vi "Poll.Main.vi"(10 "Paramaters":variant, 11 "Process":refnum<class "Process.lvclass">) -> ()   [LabVIEW 2019, in "OPC UA Client Addon Engine.lvlib"]
uses:
  OPC UA Client Addon Engine.lvlib
  <vilib>/OPCUA/NI OPC UA Client.lvlib
  Addon Shared/DataRefs.Location.ctl
  Addon Shared/OPC UA Client Addon Shared.lvlib
  <vilib>/NI/NIVS Inline Async API/_VS Inline Async API/Process/Process.lvclass
  Addon Shared/OPCConnection.Properties.ctl
  Addon Shared/Poll.ListProperties.ctl
  <vilib>/NI VeriStand/Custom Device API/Data Reference.ctl
  <vilib>/NI VeriStand/Custom Device API/Custom Device API.lvlib
  Addon Shared/Tag.WriteProperties.Info.ctl
  Addon Shared/Tags.ReadWriteRefs.ctl
  Addon Shared/Compiled.Settings.ctl
  <vilib>/NI VeriStand/Custom Device API/Custom Device Target Type.ctl
  Types/Poll.Parameters.ctl
  <vilib>/NI/NIVS Inline Async API/_Data Access Engine/Data Access Engine/Data Access Engine.lvclass
  <vilib>/NI/NIVS Inline Async API/_Data Access Engine/Data Access Engine/Methods/Write.Data.vi
  <vilib>/OPCUA/client/internal/Write Int64.vi
  <vilib>/OPCUA/client/internal/Write Int32.vi
  <vilib>/OPCUA/client/internal/Write UInt16.vi
  <vilib>/OPCUA/client/internal/Write Byte.vi
  <vilib>/OPCUA/client/internal/Write Int32 Array.vi
  <vilib>/OPCUA/client/internal/Write Bool Array.vi
  <vilib>/OPCUA/client/internal/Write SByte Array.vi
  <vilib>/OPCUA/client/internal/Write Int16.vi
  <vilib>/OPCUA/client/internal/Write SByte.vi
  <vilib>/OPCUA/client/internal/Write DateTime.vi
  <vilib>/OPCUA/client/internal/Write Bool.vi
  <vilib>/OPCUA/client/internal/Write UInt64 Array.vi
  <vilib>/OPCUA/client/internal/Write Float Array.vi
  <vilib>/OPCUA/client/internal/Write UInt64.vi
  <vilib>/OPCUA/client/internal/Write Int16 Array.vi
  <vilib>/OPCUA/client/internal/Write UInt16 Array.vi
  <vilib>/OPCUA/client/internal/Write Byte Array.vi
  <vilib>/OPCUA/client/internal/Write UInt32 Array.vi
  <vilib>/OPCUA/client/internal/Write DateTime Array.vi
  <vilib>/OPCUA/client/internal/Write Float.vi
  <vilib>/OPCUA/client/internal/Write Double Array.vi
  <vilib>/OPCUA/client/internal/Write UInt32.vi
  <vilib>/OPCUA/client/internal/Write Double.vi
  <vilib>/OPCUA/client/internal/Write Int64 Array.vi
panel:
  out "Read Code":i32
  out "Write Code":i32
  out "Read Table":variant
  out "Write Table":variant
  in  "error in (no error)":errorcluster
  out "error out":errorcluster
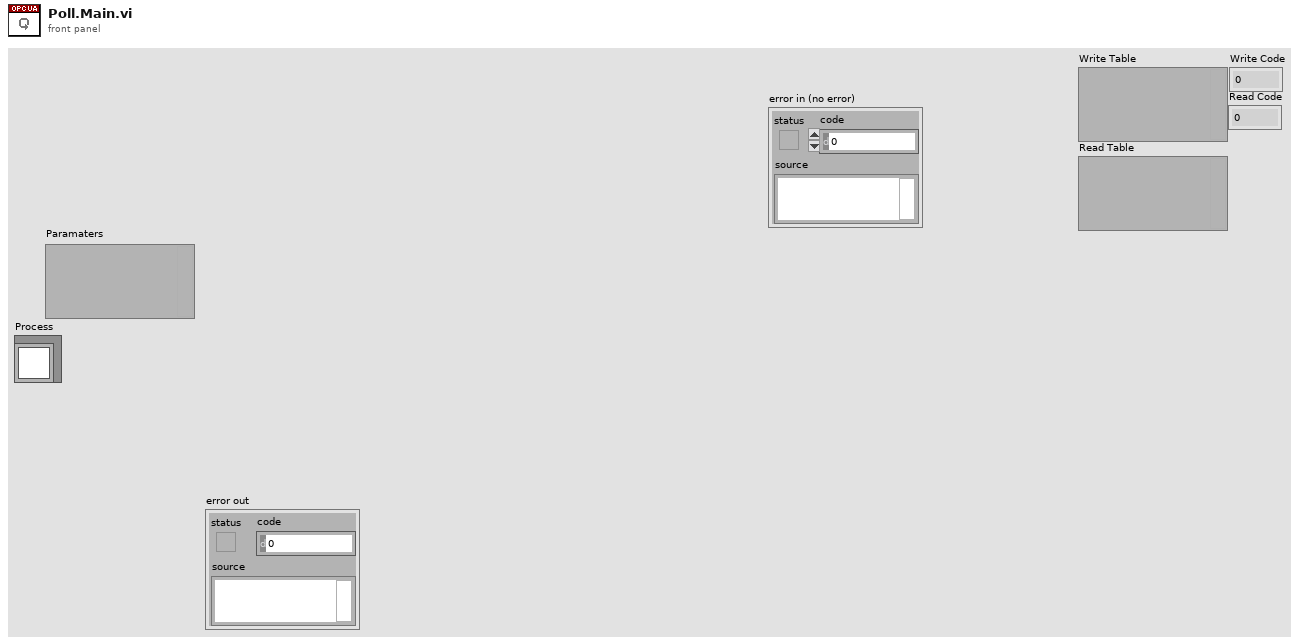
[diagram p1: front panel]
types:
  T1 = typedef "OPC UA Client Addon Engine.lvlib/Poll.Parameters.ctl" = cluster{"Name":string, "Settings":T2, "WriteData":refnum<k33>, "ReadData":refnum<k33>, "WriteUpdate":refnum<k33>, "ReadUpdate":refnum<k33>}
  T2 = typedef "OPC UA Client Addon Shared.lvlib/Compiled.Settings.ctl" = cluster{"Connection.Properties":T3, "PollEngine.Settings":T4[], "LUT":variant, "Write Locations":T5[], "TotalTags":u32, "Data Refs":T6, "Target Type":T8}
  T3 = typedef "OPC UA Client Addon Shared.lvlib/OPCConnection.Properties.ctl" = cluster{"Server IP Address":string, "Server Port":u16, "Message Mode":enum16{"None", "Sign", "Sign and Encrypt"}, "Security":enum16{"Basic256", "Basic128Rsa15"}, "User Name":string, "Password":string, "Client Certificate":path, "Server Certificate":path, "Server Certificate (RT)":path, "Client Certificate (RT)":path}
  T4 = typedef "OPC UA Client Addon Shared.lvlib/Poll.ListProperties.ctl" = cluster{"Poll Rate":dbl, "Tags":string[]}
  T5 = typedef "OPC UA Client Addon Shared.lvlib/Tag.WriteProperties.Info.ctl" = cluster{"Path":string, "Offset":i32, "Length":i32, "DataType":u32}
  T6 = typedef "OPC UA Client Addon Shared.lvlib/Tags.ReadWriteRefs.ctl" = cluster{"Read Refs":T7[], "Read Values":dbl[], "Read?":bool[], "Access":enum8{"Null", "Read", "Write", "Read&Write"}[], "Write Refs":T7[], "Write Values":dbl[], "Write?":bool[], "Write Only Location":u32, "Write? Reset":bool[]}
  T7 = typedef "Custom Device API.lvlib/Data Reference.ctl" = i32
  T8 = typedef "Custom Device API.lvlib/Custom Device Target Type.ctl" = enum16{"PharLap", "VxWorks", "Windows", "Linux_32_ARM", "Linux_x64"}
  T9 = typedef "OPC UA Client Addon Shared.lvlib/DataRefs.Location.ctl" = cluster{"Offset":i32, "Length":i32}
  T10 = typedef "OPC UA Client Addon Engine.lvlib/Poll.StateVariables.ctl" = cluster{"SubscriptionIDs":u32[], "OPCEvent":refnum<event-registration>, "Stop Ref":refnum<data-value>, "OPC UA client Ref":refnum<k21>, "Data Change":refnum<user-event>, "Process":refnum<class "Process.lvclass">, "Status Ref":T11}
  T11 = typedef "Data Access Engine.lvlib/Data Access Engine.lvclass/Write.DVR.ctl" = refnum<data-value>
  T12 = typedef "Subscription Data Change.ctl" = cluster{"node ID":T13, " value":variant, "timestamp":timestamp, "data type":T14, "status code":T15}
  T13 = typedef "NodeId.ctl" = string
  T14 = typedef "Data Type.ctl" = u16
  T15 = typedef "OPC UA StatusCode.ctl" = u32
  T16 = typedef "Subscription ID.ctl" = u32
  T17 = typedef "OPC UA Client Refnum.ctl" = refnum<k21>
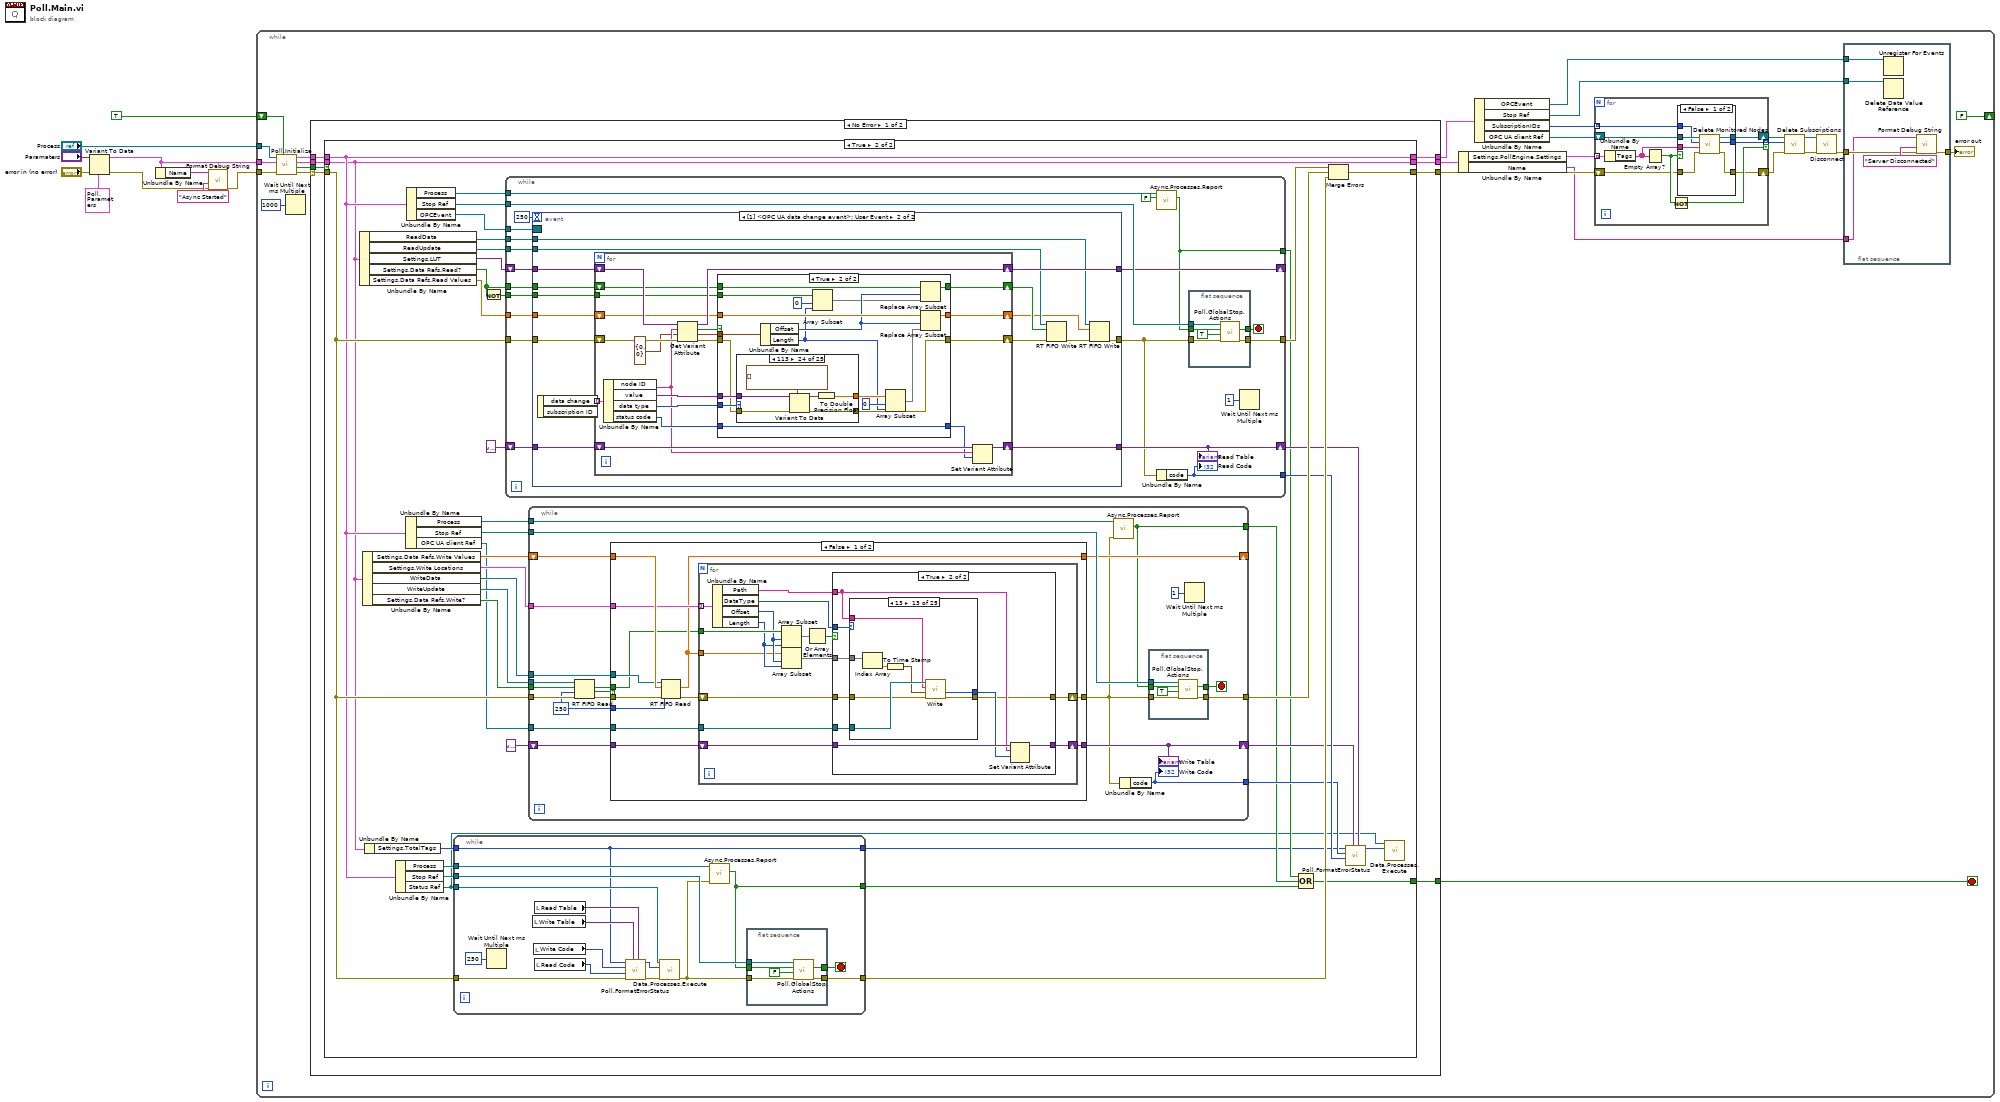
[diagram p0: block diagram]
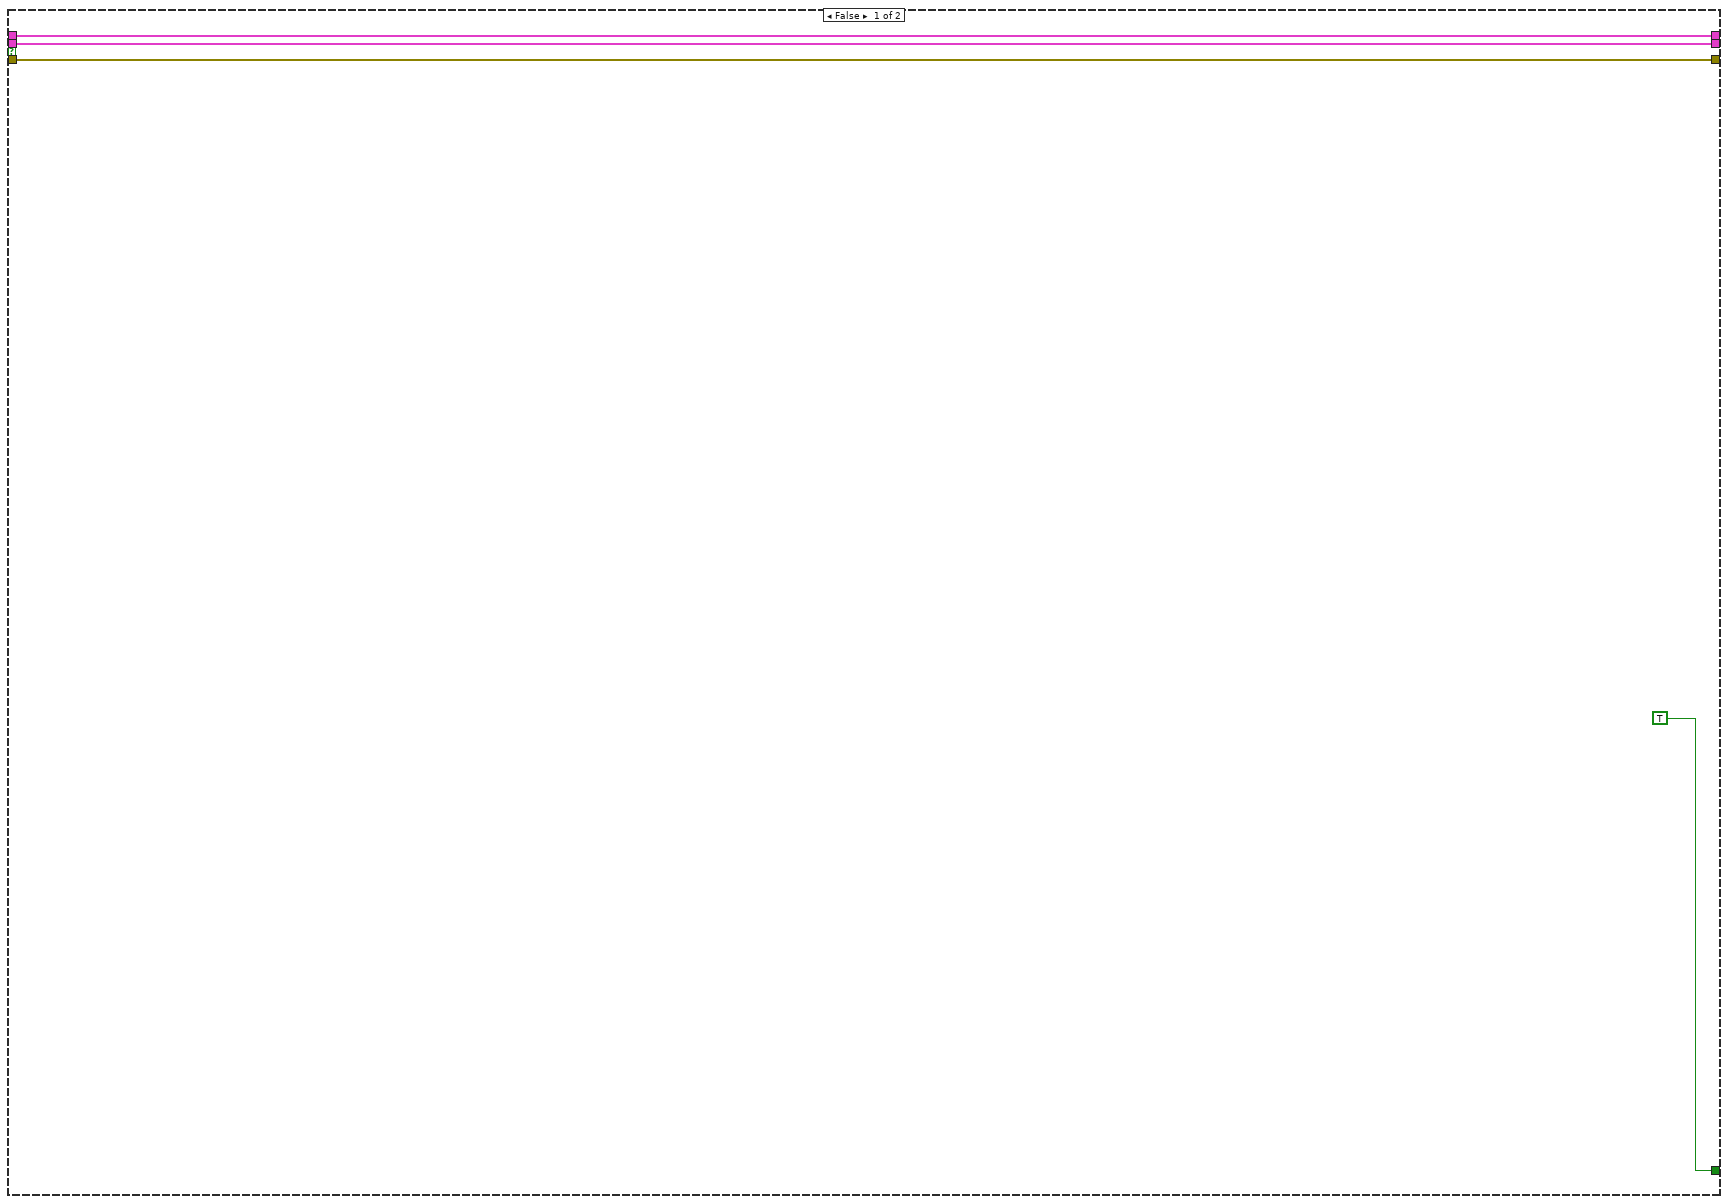
[diagram p3: hidden frame]
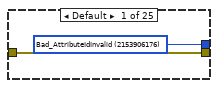
[diagram p5: hidden frame]
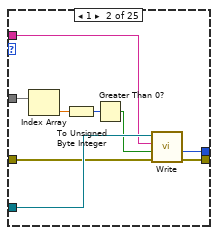
[diagram p6: hidden frame]
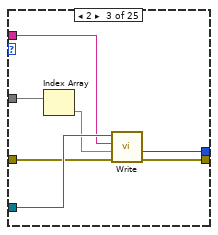
[diagram p7: hidden frame]
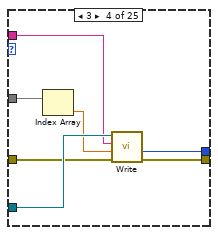
[diagram p8: hidden frame]
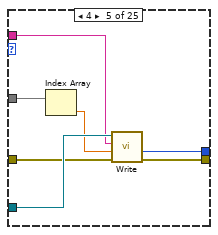
[diagram p9: hidden frame]
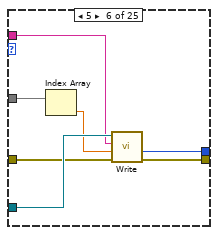
[diagram p10: hidden frame]
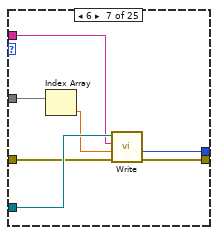
[diagram p11: hidden frame]
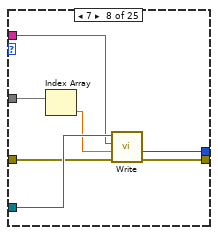
[diagram p12: hidden frame]
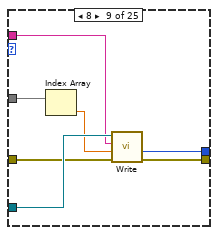
[diagram p13: hidden frame]
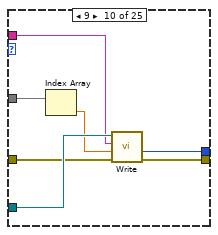
[diagram p14: hidden frame]
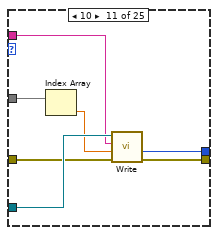
[diagram p15: hidden frame]
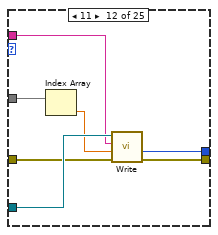
[diagram p16: hidden frame]
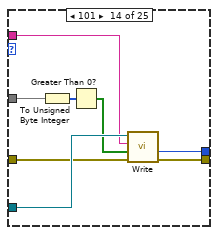
[diagram p17: hidden frame]
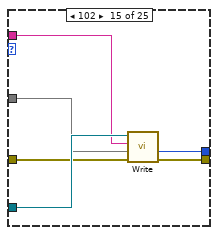
[diagram p18: hidden frame]
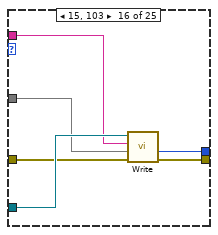
[diagram p19: hidden frame]
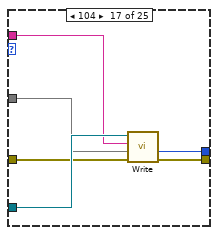
[diagram p20: hidden frame]
diagram:
  n1 = Variant To Data(error in="error in (no error)", type=T1 {"Name"="", "Settings"={"Connection.Properties"={"Server IP Address"="", "Server Port"=0, "Message Mode"=enum."None", "Security"=enum."Basic256", "User Name"="", "Password"="", "Client Certificate"=path "", "Server Certificate"=path "", "Server Certificate (RT)"=path "", "Client Certificate (RT)"=path ""}, "PollEngine.Settings"=[], "LUT"=variant, "Write Locations"=[], "TotalTags"=0, "Data Refs"={"Read Refs"=[], "Read Values"=[], "Read?"=[], "Access"=[], "Write Refs"=[], "Write Values"=[], "Write?"=[], "Write Only Location"=0, "Write? Reset"=[]}, "Target Type"=enum."PharLap"}, "WriteData"=refnum, "ReadData"=refnum, "WriteUpdate"=refnum, "ReadUpdate"=refnum} ("Parameters"), Variant="Paramaters") -> (data=w5:T1, error out=w2:errorcluster)
  n2 = Unbundle By Name(w5) -> ("Name"=w3:string)
  n3 = call "Format Debug String.vi"("error in (no error)"=w2, "State"="Async Started", "Name"=w3) -> ("error out"=w1:errorcluster)  [unwired: 8 in]
  n4 = while {
    tunnel: w1 -> [w32]
    tunnel: w5 -> [w31]
    shift-right: [FALSE] -> _
    shift-left: TRUE -> [w30]
    tunnel: "Process" -> [w27]
    stop <- w28 stop-if-true
    n5 = call "Poll.Initialize.vi"("FirstCall?"=w30, "error in (no error)"=w32, "Parameters in"=w31, "Process"=w27) -> ("error out"=w34:errorcluster, "notification"=w36:bool, "Parameters out"=w37:T1, "Settings"=w35:T10)  [unwired: 4 in]
    n6 = Wait Until Next ms Multiple(millisecond multiple=u32 1000) -> ()  [unwired: 1 out]
    n7 = case shown="No Error" w34 {
      selector: w34 -> [w67 w619]
      tunnel: [w63 w619] -> w26
      tunnel: w37 -> [w70 w623]
      tunnel: w36 -> [w69 _]
      tunnel: w35 -> [w68 w621]
      tunnel: [w65 w623] -> w25
      tunnel: [w64 w621] -> w24
      tunnel: [w66 w618] -> w28
      frame No Error {
        n8 = case shown="True" w69 {
          tunnel: w68 -> [w73 w112]
          tunnel: w67 -> [w74 w114]
          tunnel: [w74 w113] -> w63
          tunnel: w70 -> [w72 w111]
          tunnel: [w73 w112] -> w64
          tunnel: [w72 w111] -> w65
          tunnel: [TRUE w78] -> w66
          frame False {
          }
          frame True {
            n9 = Unbundle By Name(w111) -> ("ReadData"=w104:refnum<k33>, "ReadUpdate"=w91:refnum<k33>, "Settings.LUT"=w103:variant, "Settings.Data Refs.Read?"=w90:bool[], "Settings.Data Refs.Read Values"=w88:dbl[])
            n10 = Unbundle By Name(w111) -> ("Settings.Data Refs.Write Values"=w107:dbl[], "Settings.Write Locations"=w106:T5[], "WriteData"=w105:refnum<k33>, "WriteUpdate"=w93:refnum<k33>, "Settings.Data Refs.Write?"=w92:bool[])
            n11 = Unbundle By Name(w111) -> ("Settings.TotalTags"=w77:u32)
            n12 = Unbundle By Name(w112) -> ("Process"=w96:refnum<class "Process.lvclass">, "Stop Ref"=w99:refnum<data-value>, "Status Ref"=w76:T11)
            n13 = Unbundle By Name(w112) -> ("Process"=w95:refnum<class "Process.lvclass">, "Stop Ref"=w100:refnum<data-value>, "OPC UA client Ref"=w87:refnum<k21>)
            n14 = Unbundle By Name(w112) -> ("Process"=w94:refnum<class "Process.lvclass">, "Stop Ref"=w101:refnum<data-value>, "OPCEvent"=w102:refnum<event-registration>)
            n15 = while {
              tunnel: w114 -> [w130]
              tunnel: w99 -> [w129]
              tunnel: [w126] -> w98
              tunnel: w96 -> [w125]
              tunnel: [w117] -> w81
              tunnel: w76 -> [w116]
              tunnel: w77 -> [w115]
              tunnel: [w115] -> w75
              stop <- w119 stop-if-true
              n16 = Wait Until Next ms Multiple(millisecond multiple=u32 250) -> ()  [unwired: 1 out]
              n17 = local read "Write Table"() -> (w121:variant)
              n18 = local read "Write Code"() -> (w124:i32)
              n19 = local read "Read Table"() -> (w120:variant)
              n20 = local read "Read Code"() -> (w123:i32)
              n21 = call "Poll.FormatErrorStatus.vi"("Read Table"=w120, "Write Table"=w121, "error in (no error)"=w130, "Read Code"=w123, "Write Code"=w124, "TotalTags"=w115) -> ("error out"=w128:errorcluster, "ErrorStatus"=w127:u32[])  [unwired: 4 in]
              n22 = call-poly <vilib>:"Data.Processes.Execute.vi"("error in (no error)"=w128, "Values"=w127, "Ref"=w116) -> ("error out"=w118:errorcluster)  [unwired: 8 in]
              n23 = call <vilib>:"Async.Processes.Report.vi"("Error"=w118, "Process in"=w125) -> ("Stop"=w117:bool)  [unwired: 8 in, 1 out]
              n24 = flat-sequence {
                tunnel: w129 -> [w135]
                tunnel: [w134] -> w119
                tunnel: w118 -> [w133]
                tunnel: [w132] -> w126
                tunnel: w117 -> [w131]
                frame #0 {
                  n25 = call "Poll.GlobalStop.Actions.vi"("error in (no error)"=w133, "Stop on Error?"=FALSE, "Stop?"=w131, "Stop Ref"=w135) -> ("error out"=w132:errorcluster, "Latched Stop"=w134:bool)  [unwired: 5 in, 1 out]
                }
              }
            }
            n26 = Not(x=w90) -> (.not. x?=w89:bool[])
            n27 = while {
              tunnel: w102 -> [w390]
              shift-right: [w384] -> _
              shift-left: w103 -> [w387]
              tunnel: w104 -> [w379]
              tunnel: w114 -> [w388]
              tunnel: [w381] -> w97
              shift-right: [w383] -> w85
              shift-left: variant ("variant") -> [w386]
              tunnel: w101 -> [w385]
              tunnel: w94 -> [w380]
              tunnel: w91 -> [w378]
              tunnel: w90 -> [w377]
              tunnel: w89 -> [w376]
              tunnel: [w374] -> w84
              tunnel: w88 -> [w375]
              tunnel: [w371] -> w79
              stop <- w373 stop-if-true
              n28 = event shown="[1] <OPC UA data change event>: User Event" {
                selector: w390 -> [_ _]
                dyn-events: _ -> [_ _]
                timeout: 250 -> [_ _]
                tunnel: w388 -> [w399 w412]
                tunnel: [w399 w408] -> w370
                tunnel: w387 -> [w398 w414]
                tunnel: [w398 w413] -> w384
                tunnel: w386 -> [w397 w411]
                tunnel: [w397 w410] -> w383
                tunnel: w375 -> [_ w409]
                tunnel: w379 -> [_ w407]
                tunnel: w378 -> [_ w404]
                tunnel: w377 -> [_ w402]
                tunnel: w376 -> [_ w401]
                event Timeout {
                  n29 = event-data() -> ()  [unwired: 1 in, 2 out]
                }
                event User Event {
                  n30 = event-data() -> ("data change"=w415:T12[])  [unwired: 1 in, 1 out]
                  n31 = for {
                    tunnel: w415 -> [w436] mode=indexing
                    shift-right: [w432] -> w413
                    shift-left: w414 -> [w434]
                    shift-right: [w416] -> w406
                    shift-left: w412 -> [w431]
                    shift-right: [w423] -> w410
                    shift-left: w411 -> [w426]
                    shift-right: [w420] -> w400
                    shift-left: w409 -> [w421]
                    shift-right: [w418] -> w403
                    shift-left: w402 -> [w419]
                    tunnel: w401 -> [w417]
                    n32 = Unbundle By Name(w436) -> ("node ID"=w425:T13, "value"=w435:variant, "data type"=w430:T14, "status code"=w428:T15)
                    n33 = Get Variant Attribute(Variant=w434, name=w425, default value (empty Variant)=T9 {"Offset"=0, "Length"=0} ("cluster"), error in=w431) -> (duplicate Variant=w432:variant, found=w427:bool, value=w433:T9, error out=w429:errorcluster)
                    n34 = case shown="True" w427 {
                      tunnel: w435 -> [_ w458]
                      tunnel: w433 -> [_ w453]
                      tunnel: [w440 w452] -> w416
                      tunnel: w430 -> [_ w457]
                      tunnel: w429 -> [w440 w456]
                      tunnel: w428 -> [_ w455]
                      tunnel: [w439 w455] -> w424
                      tunnel: w421 -> [w438 w454]
                      tunnel: [w438 w449] -> w420
                      tunnel: w419 -> [w437 w445]
                      tunnel: [w437 w446] -> w418
                      tunnel: w417 -> [_ w442]
                      frame False {
                        w439 = u32 2153906176 items=["Good"=0, "Bad_AttributeIdInvalid"=2153906176, "Bad_BrowseDirectionInvalid"=2152529920, "Bad_BrowseNameInvalid"=2153775104, "Bad_ContentFilterInvalid"=2152202240, "Bad_ContinuationPointInvalid"=2152333312, "Bad_DataEncodingInvalid"=2151153664, "Bad_DataEncodingUnsupported"=2151219200, "Bad_EventFilterInvalid"=2152136704, "Bad_FilterNotAllowed"=2152005632, "Bad_FilterOperandInvalid"=2160132096, "Bad_HistoryOperationInvalid"=2154889216, "Bad_HistoryOperationUnsupported"=2154954752, "Bad_IndexRangeInvalid"=2151022592, "Bad_IndexRangeNoData"=2151088128, "Bad_MonitoredItemFilterInvalid"=2151874560, "Bad_MonitoredItemFilterUnsupported"=2151940096, "Bad_MonitoredItemIdInvalid"=2151809024, "Bad_MonitoringModeInvalid"=2151743488, "Bad_NoCommunication"=2150694912, "Bad_NoContinuationPoints"=2152398848, "Bad_NodeClassInvalid"=2153709568, "Bad_NodeIdInvalid"=2150825984, "Bad_NodeIdUnknown"=2150891520, "Bad_NoDeleteRights"=2154364928, "Bad_NodeNotInView"=2152595456, "Bad_NotFound"=2151546880, "Bad_NotImplemented"=2151677952, "Bad_NotReadable"=2151284736, "Bad_NotSupported"=2151481344, "Bad_NotWritable"=2151350272, "Bad_ObjectDeleted"=2151612416, "Bad_OutOfRange"=2151415808, "Bad_ReferenceTypeIdInvalid"=2152464384, "Bad_SourceNodeIdInvalid"=2154037248, "Bad_StructureMissing"=2152071168, "Bad_TargetNodeIdInvalid"=2154102784, "Bad_TypeDefinitionInvalid"=2153971712, "Bad_TypeMismatch"=2155085824, "Bad_WaitingForInitialData"=2150760448] ("status")
                      }
                      frame True {
                        n35 = case shown="113" w457 {
                          tunnel: w458 -> [w466 w473 w480 w487 w494 w501 w508 w515 w522 w529 w536 w543 w550 w556 w562 w568 w574 w580 w586 w592 w598 w604 w610 w616 _]
                          tunnel: w456 -> [w465 w472 w479 w486 w493 w500 w507 w514 w521 w528 w535 w542 w549 w555 w561 w567 w573 w579 w585 w591 w597 w603 w609 w615 w617]
                          tunnel: [w464 w471 w478 w485 w492 w499 w506 w513 w520 w527 w534 w541 w548 w554 w560 w566 w572 w578 w584 w590 w596 w602 w608 w614 w617] -> w452
                          tunnel: [w459 w468 w475 w482 w489 w496 w503 w510 w517 w524 w531 w538 w544 w552 w558 w564 w570 w576 w582 w588 w594 w600 w606 w612 _] -> w451
                          frame 1 {
                            n36 = Variant To Data(error in=w465, type=FALSE, Variant=w466) -> (data=w462:bool, error out=w464:errorcluster)
                            n37 = Boolean To (0,1)(Boolean=w462) -> (0, 1=w461:i16)
                            n38 = To Double Precision Float(number=w461) -> (double precision float=w460:dbl)
                            n39 = Build Array(w460) -> (w459:dbl[])
                          }
                          frame 2 {
                            n40 = Variant To Data(error in=w472, type=i8 0, Variant=w473) -> (data=w467:i8, error out=w471:errorcluster)
                            n41 = To Double Precision Float(number=w467) -> (double precision float=w469:dbl)
                            n42 = Build Array(w469) -> (w468:dbl[])
                          }
                          frame 3 {
                            n43 = Variant To Data(error in=w479, type=u8 0, Variant=w480) -> (data=w474:u8, error out=w478:errorcluster)
                            n44 = To Double Precision Float(number=w474) -> (double precision float=w476:dbl)
                            n45 = Build Array(w476) -> (w475:dbl[])
                          }
                          frame 4 {
                            n46 = Variant To Data(error in=w486, type=i16 0, Variant=w487) -> (data=w481:i16, error out=w485:errorcluster)
                            n47 = To Double Precision Float(number=w481) -> (double precision float=w483:dbl)
                            n48 = Build Array(w483) -> (w482:dbl[])
                          }
                          frame 5 {
                            n49 = Variant To Data(error in=w493, type=u16 0, Variant=w494) -> (data=w488:u16, error out=w492:errorcluster)
                            n50 = To Double Precision Float(number=w488) -> (double precision float=w490:dbl)
                            n51 = Build Array(w490) -> (w489:dbl[])
                          }
                          frame 6 {
                            n52 = Variant To Data(error in=w500, type=0, Variant=w501) -> (data=w495:i32, error out=w499:errorcluster)
                            n53 = To Double Precision Float(number=w495) -> (double precision float=w497:dbl)
                            n54 = Build Array(w497) -> (w496:dbl[])
                          }
                          frame 7 {
                            n55 = Variant To Data(error in=w507, type=u32 0, Variant=w508) -> (data=w502:u32, error out=w506:errorcluster)
                            n56 = To Double Precision Float(number=w502) -> (double precision float=w504:dbl)
                            n57 = Build Array(w504) -> (w503:dbl[])
                          }
                          frame 8 {
                            n58 = Variant To Data(error in=w514, type=i64 0, Variant=w515) -> (data=w509:i64, error out=w513:errorcluster)
                            n59 = To Double Precision Float(number=w509) -> (double precision float=w511:dbl)
                            n60 = Build Array(w511) -> (w510:dbl[])
                          }
                          frame 9 {
                            n61 = Variant To Data(error in=w521, type=u64 0, Variant=w522) -> (data=w516:u64, error out=w520:errorcluster)
                            n62 = To Double Precision Float(number=w516) -> (double precision float=w518:dbl)
                            n63 = Build Array(w518) -> (w517:dbl[])
                          }
                          frame 10 {
                            n64 = Variant To Data(error in=w528, type=sgl 0.0, Variant=w529) -> (data=w523:sgl, error out=w527:errorcluster)
                            n65 = To Double Precision Float(number=w523) -> (double precision float=w525:dbl)
                            n66 = Build Array(w525) -> (w524:dbl[])
                          }
                          frame 11 {
                            n67 = Variant To Data(error in=w535, type=0.0, Variant=w536) -> (data=w530:dbl, error out=w534:errorcluster)
                            n68 = To Double Precision Float(number=w530) -> (double precision float=w532:dbl)
                            n69 = Build Array(w532) -> (w531:dbl[])
                          }
                          frame 13 {
                            n70 = Variant To Data(error in=w542, type=timestamp(0 s since 1904-01-01), Variant=w543) -> (data=w537:timestamp, error out=w541:errorcluster)
                            n71 = To Double Precision Float(number=w537) -> (double precision float=w539:dbl)
                            n72 = Build Array(w539) -> (w538:dbl[])
                          }
                          frame 101 {
                            n73 = Variant To Data(error in=w549, type=bool[] [], Variant=w550) -> (data=w547:bool[], error out=w548:errorcluster)
                            n74 = Boolean To (0,1)(Boolean=w547) -> (0, 1=w546:i16[])
                            n75 = To Double Precision Float(number=w546) -> (double precision float=w544:dbl[])
                          }
                          frame 102 {
                            n76 = Variant To Data(error in=w555, type=i8[] [], Variant=w556) -> (data=w551:i8[], error out=w554:errorcluster)
                            n77 = To Double Precision Float(number=w551) -> (double precision float=w552:dbl[])
                          }
                          frame 15, 103 {
                            n78 = Variant To Data(error in=w561, type=u8[] [], Variant=w562) -> (data=w557:u8[], error out=w560:errorcluster)
                            n79 = To Double Precision Float(number=w557) -> (double precision float=w558:dbl[])
                          }
                          frame 104 {
                            n80 = Variant To Data(error in=w567, type=i16[] [], Variant=w568) -> (data=w563:i16[], error out=w566:errorcluster)
                            n81 = To Double Precision Float(number=w563) -> (double precision float=w564:dbl[])
                          }
                          frame 105 {
                            n82 = Variant To Data(error in=w573, type=u16[] [], Variant=w574) -> (data=w569:u16[], error out=w572:errorcluster)
                            n83 = To Double Precision Float(number=w569) -> (double precision float=w570:dbl[])
                          }
                          frame 106 {
                            n84 = Variant To Data(error in=w579, type=i32[] [], Variant=w580) -> (data=w575:i32[], error out=w578:errorcluster)
                            n85 = To Double Precision Float(number=w575) -> (double precision float=w576:dbl[])
                          }
                          frame 107 {
                            n86 = Variant To Data(error in=w585, type=u32[] [], Variant=w586) -> (data=w581:u32[], error out=w584:errorcluster)
                            n87 = To Double Precision Float(number=w581) -> (double precision float=w582:dbl[])
                          }
                          frame 108 {
                            n88 = Variant To Data(error in=w591, type=i64[] [], Variant=w592) -> (data=w587:i64[], error out=w590:errorcluster)
                            n89 = To Double Precision Float(number=w587) -> (double precision float=w588:dbl[])
                          }
                          frame 109 {
                            n90 = Variant To Data(error in=w597, type=u64[] [], Variant=w598) -> (data=w593:u64[], error out=w596:errorcluster)
                            n91 = To Double Precision Float(number=w593) -> (double precision float=w594:dbl[])
                          }
                          frame 110 {
                            n92 = Variant To Data(error in=w603, type=sgl[] [], Variant=w604) -> (data=w599:sgl[], error out=w602:errorcluster)
                            n93 = To Double Precision Float(number=w599) -> (double precision float=w600:dbl[])
                          }
                          frame 111 {
                            n94 = Variant To Data(error in=w609, type=dbl[] [], Variant=w610) -> (data=w605:dbl[], error out=w608:errorcluster)
                            n95 = To Double Precision Float(number=w605) -> (double precision float=w606:dbl[])
                          }
                          frame 113 {
                            n96 = Variant To Data(error in=w615, type=timestamp[] [], Variant=w616) -> (data=w611:timestamp[], error out=w614:errorcluster)
                            n97 = To Double Precision Float(number=w611) -> (double precision float=w612:dbl[])
                          }
                          frame Default {
                          }
                        }
                        n98 = Unbundle By Name(w453) -> ("Offset"=w448:i32, "Length"=w444:i32)
                        n99 = Array Subset(array=w442, index=0, length=w444) -> (w441:bool[])
                        n100 = Array Subset(array=w451, index=0, length=w444) -> (w450:dbl[])
                        n101 = Replace Array Subset(array=w445, new element=w441, index=w448) -> (w446:bool[])
                        n102 = Replace Array Subset(array=w454, new element=w450, index=w448) -> (w449:dbl[])
                      }
                    }
                    n103 = Set Variant Attribute(Variant=w426, name=w425, value=w424) -> (Variant out=w423:variant)  [unwired: 1 in, 2 out]
                  }
                  n104 = RT FIFO Write(0:w404, 1:w403, 3:w406) -> (11:w405:errorcluster)  [unwired: 2 in, 3 out]
                  n105 = RT FIFO Write(0:w407, 1:w400, 3:w405) -> (11:w408:errorcluster)  [unwired: 2 in, 3 out]
                }
              }
              "Read Table" <- w383
              n106 = call <vilib>:"Async.Processes.Report.vi"("Stop Async on Error?"=FALSE ("Stop on Error?"), "Process in"=w380) -> ("Stop"=w371:bool)  [unwired: 8 in, 1 out]
              n107 = Unbundle By Name(w370) -> ("code"=w374:i32)
              "Read Code" <- w374
              n108 = flat-sequence {
                tunnel: w370 -> [w396]
                tunnel: w385 -> [w394]
                tunnel: [w393] -> w381
                tunnel: [w392] -> w373
                tunnel: w371 -> [w391]
                frame #0 {
                  n109 = call "Poll.GlobalStop.Actions.vi"("error in (no error)"=w396, "Stop on Error?"=TRUE, "Stop?"=w391, "Stop Ref"=w394) -> ("error out"=w393:errorcluster, "Latched Stop"=w392:bool)  [unwired: 5 in, 1 out]
                }
              }
              n110 = Wait Until Next ms Multiple(millisecond multiple=u32 1) -> ()  [unwired: 1 out]
            }
            n111 = while {
              tunnel: w106 -> [w157]
              shift-right: [w150] -> _
              shift-left: w107 -> [w158]
              tunnel: w105 -> [w155]
              tunnel: w114 -> [w149]
              tunnel: [w151] -> w108
              shift-right: [w154] -> w82
              shift-left: variant ("variant") -> [w153]
              tunnel: w100 -> [w152]
              tunnel: w95 -> [w139]
              tunnel: w93 -> [w147]
              tunnel: w92 -> [w146]
              tunnel: [w141] -> w83
              tunnel: [w138] -> w80
              tunnel: w87 -> [w156]
              stop <- w140 stop-if-true
              w145 = 250 ("timeout in ms (0)")
              n112 = RT FIFO Read(0:w147, 1:w146, 2:w145, 3:w149) -> (9:w144:bool[], 10:w143:bool, 11:w148:errorcluster)  [unwired: 2 out]
              n113 = case shown="False" w143 {
                tunnel: w158 -> [w175 w369]
                tunnel: w157 -> [w174 _]
                tunnel: w156 -> [w173 _]
                tunnel: w155 -> [w172 _]
                tunnel: [w171 w367] -> w154
                tunnel: w153 -> [w170 w367]
                tunnel: [w169 w368] -> w137
                tunnel: [w168 w369] -> w150
                tunnel: w148 -> [w167 w368]
                tunnel: w145 -> [w166 _]
                tunnel: w144 -> [w165 _]
                frame False {
                  n114 = RT FIFO Read(0:w172, 1:w175, 2:w166, 3:w167) -> (9:w168:dbl[], 11:w176:errorcluster)  [unwired: 3 out]
                  n115 = for {
                    tunnel: w165 -> [w188]
                    tunnel: w174 -> [w186] mode=indexing
                    shift-right: [w190] -> w169
                    shift-left: w176 -> [w189]
                    tunnel: w168 -> [w182]
                    shift-right: [w180] -> w171
                    shift-left: w170 -> [w181]
                    tunnel: w173 -> [w191]
                    n116 = Unbundle By Name(w186) -> ("Path"=w179:string, "DataType"=w183:u32, "Offset"=w185:i32, "Length"=w184:i32)
                    n117 = Array Subset(array=w188, index=w185, length=w184) -> (w177:bool[])
                    n118 = Array Subset(array=w182, index=w185, length=w184) -> (w187:dbl[])
                    n119 = Or Array Elements(Boolean array=w177) -> (logical OR=w178:bool)
                    n120 = case shown="True" w178 {
                      tunnel: w191 -> [_ w202]
                      tunnel: [w193 w194] -> w190
                      tunnel: w189 -> [w193 w201]
                      tunnel: w179 -> [_ w195]
                      tunnel: w187 -> [_ w200]
                      tunnel: w183 -> [_ w199]
                      tunnel: w181 -> [w192 w198]
                      tunnel: [w192 w196] -> w180
                      frame False {
                      }
                      frame True {
                        n121 = case shown="13" w199 {
                          tunnel: w202 -> [_ w213 w220 w227 w234 w241 w248 w255 w262 w269 w276 w283 w291 w299 w305 w311 w317 w323 w329 w335 w341 w347 w353 w359 w366]
                          tunnel: [w204 w212 w219 w226 w233 w240 w247 w254 w261 w268 w275 w282 w290 w298 w304 w310 w316 w322 w328 w334 w340 w346 w352 w358 w365] -> w194
                          tunnel: w201 -> [w204 w211 w218 w225 w232 w239 w246 w253 w260 w267 w274 w281 w289 w297 w303 w309 w315 w321 w327 w333 w339 w345 w351 w357 w364]
                          tunnel: w200 -> [_ w209 w216 w223 w230 w237 w244 w251 w258 w265 w272 w279 w287 w295 w302 w308 w314 w320 w326 w332 w338 w344 w350 w356 w363]
                          tunnel: w195 -> [_ w206 w215 w222 w229 w236 w243 w250 w257 w264 w271 w278 w285 w293 w301 w307 w313 w319 w325 w331 w337 w343 w349 w355 w362]
                          tunnel: [w203 w205 w214 w221 w228 w235 w242 w249 w256 w263 w270 w277 w284 w292 w300 w306 w312 w318 w324 w330 w336 w342 w348 w354 w360] -> w197
                          frame Default {
                            w203 = u32 2153906176 items=["Good"=0, "Bad_AttributeIdInvalid"=2153906176, "Bad_BrowseDirectionInvalid"=2152529920, "Bad_BrowseNameInvalid"=2153775104, "Bad_ContentFilterInvalid"=2152202240, "Bad_ContinuationPointInvalid"=2152333312, "Bad_DataEncodingInvalid"=2151153664, "Bad_DataEncodingUnsupported"=2151219200, "Bad_EventFilterInvalid"=2152136704, "Bad_FilterNotAllowed"=2152005632, "Bad_FilterOperandInvalid"=2160132096, "Bad_HistoryOperationInvalid"=2154889216, "Bad_HistoryOperationUnsupported"=2154954752, "Bad_IndexRangeInvalid"=2151022592, "Bad_IndexRangeNoData"=2151088128, "Bad_MonitoredItemFilterInvalid"=2151874560, "Bad_MonitoredItemFilterUnsupported"=2151940096, "Bad_MonitoredItemIdInvalid"=2151809024, "Bad_MonitoringModeInvalid"=2151743488, "Bad_NoCommunication"=2150694912, "Bad_NoContinuationPoints"=2152398848, "Bad_NodeClassInvalid"=2153709568, "Bad_NodeIdInvalid"=2150825984, "Bad_NodeIdUnknown"=2150891520, "Bad_NoDeleteRights"=2154364928, "Bad_NodeNotInView"=2152595456, "Bad_NotFound"=2151546880, "Bad_NotImplemented"=2151677952, "Bad_NotReadable"=2151284736, "Bad_NotSupported"=2151481344, "Bad_NotWritable"=2151350272, "Bad_ObjectDeleted"=2151612416, "Bad_OutOfRange"=2151415808, "Bad_ReferenceTypeIdInvalid"=2152464384, "Bad_SourceNodeIdInvalid"=2154037248, "Bad_StructureMissing"=2152071168, "Bad_TargetNodeIdInvalid"=2154102784, "Bad_TypeDefinitionInvalid"=2153971712, "Bad_TypeMismatch"=2155085824, "Bad_WaitingForInitialData"=2150760448] ("status")
                          }
                          frame 1 {
                            n122 = Index Array(array=w209) -> (element=w210:dbl)  [unwired: 1 in]
                            n123 = To Unsigned Byte Integer(number=w210) -> (unsigned 8bit integer=w207:u8)
                            n124 = Greater Than 0?(x=w207) -> (x > 0?=w208:bool)
                            n125 = call-poly <vilib>:"Write.vi"("error in (no error)"=w211, "value"=w208, "node ID"=w206, "OPC UA client refnum in"=w213) -> ("error out"=w212:errorcluster, "status"=w205:T15)  [unwired: 5 in, 1 out]
                          }
                          frame 2 {
                            n126 = Index Array(array=w216) -> (element=w217:dbl)  [unwired: 1 in]
                            n127 = call-poly <vilib>:"Write.vi"("error in (no error)"=w218, "value"=w217, "node ID"=w215, "OPC UA client refnum in"=w220) -> ("error out"=w219:errorcluster, "status"=w214:T15)  [unwired: 5 in, 1 out]
                          }
                          frame 3 {
                            n128 = Index Array(array=w223) -> (element=w224:dbl)  [unwired: 1 in]
                            n129 = call-poly <vilib>:"Write.vi"("error in (no error)"=w225, "value"=w224, "node ID"=w222, "OPC UA client refnum in"=w227) -> ("error out"=w226:errorcluster, "status"=w221:T15)  [unwired: 5 in, 1 out]
                          }
                          frame 4 {
                            n130 = Index Array(array=w230) -> (element=w231:dbl)  [unwired: 1 in]
                            n131 = call-poly <vilib>:"Write.vi"("error in (no error)"=w232, "value"=w231, "node ID"=w229, "OPC UA client refnum in"=w234) -> ("error out"=w233:errorcluster, "status"=w228:T15)  [unwired: 5 in, 1 out]
                          }
                          frame 5 {
                            n132 = Index Array(array=w237) -> (element=w238:dbl)  [unwired: 1 in]
                            n133 = call-poly <vilib>:"Write.vi"("error in (no error)"=w239, "value"=w238, "node ID"=w236, "OPC UA client refnum in"=w241) -> ("error out"=w240:errorcluster, "status"=w235:T15)  [unwired: 5 in, 1 out]
                          }
                          frame 6 {
                            n134 = Index Array(array=w244) -> (element=w245:dbl)  [unwired: 1 in]
                            n135 = call-poly <vilib>:"Write.vi"("error in (no error)"=w246, "value"=w245, "node ID"=w243, "OPC UA client refnum in"=w248) -> ("error out"=w247:errorcluster, "status"=w242:T15)  [unwired: 5 in, 1 out]
                          }
                          frame 7 {
                            n136 = Index Array(array=w251) -> (element=w252:dbl)  [unwired: 1 in]
                            n137 = call-poly <vilib>:"Write.vi"("error in (no error)"=w253, "value"=w252, "node ID"=w250, "OPC UA client refnum in"=w255) -> ("error out"=w254:errorcluster, "status"=w249:T15)  [unwired: 5 in, 1 out]
                          }
                          frame 8 {
                            n138 = Index Array(array=w258) -> (element=w259:dbl)  [unwired: 1 in]
                            n139 = call-poly <vilib>:"Write.vi"("error in (no error)"=w260, "value"=w259, "node ID"=w257, "OPC UA client refnum in"=w262) -> ("error out"=w261:errorcluster, "status"=w256:T15)  [unwired: 5 in, 1 out]
                          }
                          frame 9 {
                            n140 = Index Array(array=w265) -> (element=w266:dbl)  [unwired: 1 in]
                            n141 = call-poly <vilib>:"Write.vi"("error in (no error)"=w267, "value"=w266, "node ID"=w264, "OPC UA client refnum in"=w269) -> ("error out"=w268:errorcluster, "status"=w263:T15)  [unwired: 5 in, 1 out]
                          }
                          frame 10 {
                            n142 = Index Array(array=w272) -> (element=w273:dbl)  [unwired: 1 in]
                            n143 = call-poly <vilib>:"Write.vi"("error in (no error)"=w274, "value"=w273, "node ID"=w271, "OPC UA client refnum in"=w276) -> ("error out"=w275:errorcluster, "status"=w270:T15)  [unwired: 5 in, 1 out]
                          }
                          frame 11 {
                            n144 = Index Array(array=w279) -> (element=w280:dbl)  [unwired: 1 in]
                            n145 = call-poly <vilib>:"Write.vi"("error in (no error)"=w281, "value"=w280, "node ID"=w278, "OPC UA client refnum in"=w283) -> ("error out"=w282:errorcluster, "status"=w277:T15)  [unwired: 5 in, 1 out]
                          }
                          frame 13 {
                            n146 = Index Array(array=w287) -> (element=w288:dbl)  [unwired: 1 in]
                            n147 = To Time Stamp(1:w288) -> (0:w286:timestamp)
                            n148 = call-poly <vilib>:"Write.vi"("error in (no error)"=w289, "value"=w286, "node ID"=w285, "OPC UA client refnum in"=w291) -> ("error out"=w290:errorcluster, "status"=w284:T15)  [unwired: 5 in, 1 out]
                          }
                          frame 101 {
                            n149 = To Unsigned Byte Integer(number=w295) -> (unsigned 8bit integer=w296:u8[])
                            n150 = Greater Than 0?(x=w296) -> (x > 0?=w294:bool[])
                            n151 = call-poly <vilib>:"Write.vi"("error in (no error)"=w297, "values"=w294, "node ID"=w293, "OPC UA client refnum in"=w299) -> ("error out"=w298:errorcluster, "status"=w292:T15)  [unwired: 5 in, 1 out]
                          }
                          frame 102 {
                            n152 = call-poly <vilib>:"Write.vi"("error in (no error)"=w303, "values"=w302, "node ID"=w301, "OPC UA client refnum in"=w305) -> ("error out"=w304:errorcluster, "status"=w300:T15)  [unwired: 5 in, 1 out]
                          }
                          frame 15, 103 {
                            n153 = call-poly <vilib>:"Write.vi"("error in (no error)"=w309, "values"=w308, "node ID"=w307, "OPC UA client refnum in"=w311) -> ("error out"=w310:errorcluster, "status"=w306:T15)  [unwired: 5 in, 1 out]
                          }
                          frame 104 {
                            n154 = call-poly <vilib>:"Write.vi"("error in (no error)"=w315, "values"=w314, "node ID"=w313, "OPC UA client refnum in"=w317) -> ("error out"=w316:errorcluster, "status"=w312:T15)  [unwired: 5 in, 1 out]
                          }
                          frame 105 {
                            n155 = call-poly <vilib>:"Write.vi"("error in (no error)"=w321, "values"=w320, "node ID"=w319, "OPC UA client refnum in"=w323) -> ("error out"=w322:errorcluster, "status"=w318:T15)  [unwired: 5 in, 1 out]
                          }
                          frame 106 {
                            n156 = call-poly <vilib>:"Write.vi"("error in (no error)"=w327, "values"=w326, "node ID"=w325, "OPC UA client refnum in"=w329) -> ("error out"=w328:errorcluster, "status"=w324:T15)  [unwired: 5 in, 1 out]
                          }
                          frame 107 {
                            n157 = call-poly <vilib>:"Write.vi"("error in (no error)"=w333, "values"=w332, "node ID"=w331, "OPC UA client refnum in"=w335) -> ("error out"=w334:errorcluster, "status"=w330:T15)  [unwired: 5 in, 1 out]
                          }
                          frame 108 {
                            n158 = call-poly <vilib>:"Write.vi"("error in (no error)"=w339, "values"=w338, "node ID"=w337, "OPC UA client refnum in"=w341) -> ("error out"=w340:errorcluster, "status"=w336:T15)  [unwired: 5 in, 1 out]
                          }
                          frame 109 {
                            n159 = call-poly <vilib>:"Write.vi"("error in (no error)"=w345, "values"=w344, "node ID"=w343, "OPC UA client refnum in"=w347) -> ("error out"=w346:errorcluster, "status"=w342:T15)  [unwired: 5 in, 1 out]
                          }
                          frame 110 {
                            n160 = call-poly <vilib>:"Write.vi"("error in (no error)"=w351, "values"=w350, "node ID"=w349, "OPC UA client refnum in"=w353) -> ("error out"=w352:errorcluster, "status"=w348:T15)  [unwired: 5 in, 1 out]
                          }
                          frame 111 {
                            n161 = call-poly <vilib>:"Write.vi"("error in (no error)"=w357, "values"=w356, "node ID"=w355, "OPC UA client refnum in"=w359) -> ("error out"=w358:errorcluster, "status"=w354:T15)  [unwired: 5 in, 1 out]
                          }
                          frame 113 {
                            n162 = To Time Stamp(1:w363) -> (0:w361:timestamp[])
                            n163 = call-poly <vilib>:"Write.vi"("error in (no error)"=w364, "values"=w361, "node ID"=w362, "OPC UA client refnum in"=w366) -> ("error out"=w365:errorcluster, "status"=w360:T15)  [unwired: 5 in, 1 out]
                          }
                        }
                        n164 = Set Variant Attribute(Variant=w198, name=w195, value=w197) -> (Variant out=w196:variant)  [unwired: 1 in, 2 out]
                      }
                    }
                  }
                }
                frame True {
                }
              }
              "Write Table" <- w154
              n165 = call <vilib>:"Async.Processes.Report.vi"("Error"=w137, "Process in"=w139) -> ("Stop"=w138:bool)  [unwired: 8 in, 1 out]
              n166 = Unbundle By Name(w137) -> ("code"=w141:i32)
              "Write Code" <- w141
              n167 = flat-sequence {
                tunnel: w137 -> [w164]
                tunnel: w152 -> [w163]
                tunnel: [w161] -> w151
                tunnel: [w160] -> w140
                tunnel: w138 -> [w159]
                frame #0 {
                  n168 = call "Poll.GlobalStop.Actions.vi"("error in (no error)"=w164, "Stop on Error?"=TRUE, "Stop?"=w159, "Stop Ref"=w163) -> ("error out"=w161:errorcluster, "Latched Stop"=w160:bool)  [unwired: 5 in, 1 out]
                }
              }
              n169 = Wait Until Next ms Multiple(millisecond multiple=u32 1) -> ()  [unwired: 1 out]
            }
            n170 = Compound Arithmetic op=OR(w79, w80, w81) -> (w78:bool)
            n171 = Merge Errors(w97, w108, w98) -> (w113:errorcluster)
            n172 = call "Poll.FormatErrorStatus.vi"("Read Table"=w85, "Write Table"=w82, "Read Code"=w84, "Write Code"=w83, "TotalTags"=w75) -> ("ErrorStatus"=w86:u32[])  [unwired: 5 in, 1 out]
            n173 = call-poly <vilib>:"Data.Processes.Execute.vi"("Values"=w86, "Ref"=w76) -> ()  [unwired: 9 in, 1 out]
          }
        }
      }
      frame Error {
        n174 = Unbundle By Name(w621) -> ("Process"=w620:refnum<class "Process.lvclass">)
        n175 = call <vilib>:"Async.Processes.Report.vi"("Error"=w619, "Stop Async on Error?"=FALSE ("Stop on Error?"), "Process in"=w620) -> ("Stop"=w618:bool)  [unwired: 7 in, 1 out]
      }
    }
    n176 = Unbundle By Name(w25) -> ("Settings.PollEngine.Settings"=w22:T4[], "Name"=w11:string)
    n177 = Unbundle By Name(w24) -> ("OPCEvent"=w18:refnum<event-registration>, "Stop Ref"=w19:refnum<data-value>, "SubscriptionIDs"=w21:u32[], "OPC UA client Ref"=w14:refnum<k21>)
    n178 = for {
      tunnel: w21 -> [w53] mode=indexing
      tunnel: w22 -> [w52] mode=indexing
      tunnel: [w50] -> w20 mode=indexing if=w48
      shift-right: [w46] -> w17
      shift-left: w26 -> [w47]
      shift-right: [w44] -> w13
      shift-left: w14 -> [w45]
      n179 = Unbundle By Name(w52) -> ("Tags"=w51:string[])
      n180 = Empty Array?(array=w51) -> (empty?=w49:bool)
      n181 = Not(x=w49) -> (.not. x?=w48:bool)
      n182 = case shown="False" w49 {
        tunnel: w45 -> [w60 w61]
        tunnel: w53 -> [w59 _]
        tunnel: w51 -> [w58 _]
        tunnel: [w57 _] -> w50
        tunnel: w47 -> [w56 w62]
        tunnel: [w55 w62] -> w46
        tunnel: [w54 w61] -> w44
        frame False {
          n183 = call <vilib>:"Delete Monitored Nodes.vi"("error in (no error)"=w56, "node IDs"=w58, "subscription ID in"=w59, "OPC UA client refnum in"=w60) -> ("error out"=w55:errorcluster, "subscription ID out"=w57:T16, "OPC UA client refnum out"=w54:T17)  [unwired: 3 in, 2 out]
        }
        frame True {
        }
      }
    }
    n184 = call <vilib>:"Delete Subscriptions.vi"("error in (no error)"=w17, "subscription IDs"=w20, "OPC UA client refnum in"=w13) -> ("error out"=w16:errorcluster, "OPC UA client refnum out"=w23:T17)  [unwired: 6 in, 1 out]
    n185 = call <vilib>:"Disconnect.vi"("error in (no error)"=w16, "OPC UA client refnum in"=w23) -> ("error out"=w15:errorcluster)  [unwired: 9 in]
    n186 = flat-sequence {
      tunnel: w19 -> [w43]
      tunnel: w18 -> [w42]
      tunnel: w15 -> [w40]
      tunnel: [w39] -> w12
      tunnel: w11 -> [w38]
      frame #0 {
        n187 = Unregister For Events(event registration refnum=w42) -> ()  [unwired: 1 in, 1 out]
        n188 = Delete Data Value Reference(data value reference=w43) -> ()  [unwired: 1 in, 2 out]
        n189 = call "Format Debug String.vi"("error in (no error)"=w40, "State"="Server Disconnected", "Name"=w38) -> ("error out"=w39:errorcluster)  [unwired: 8 in]
      }
    }
    "error out" <- w12
  }
